vi "read_session.vi"(8 "error in (no error)":errorcluster caption="entrée d'erreur (pas d'erreur)", 11 "Python en entrée":refnum<class "Python.lvclass">) -> (0 "error out":errorcluster caption="sortie d'erreur", 2 "session":refnum<k35>, 3 "Python en sortie":refnum<class "Python.lvclass">)   [LabVIEW 2020, in "Python.lvclass"]
uses:
  Python.lvclass
  Python.lvclass/Python.ctl
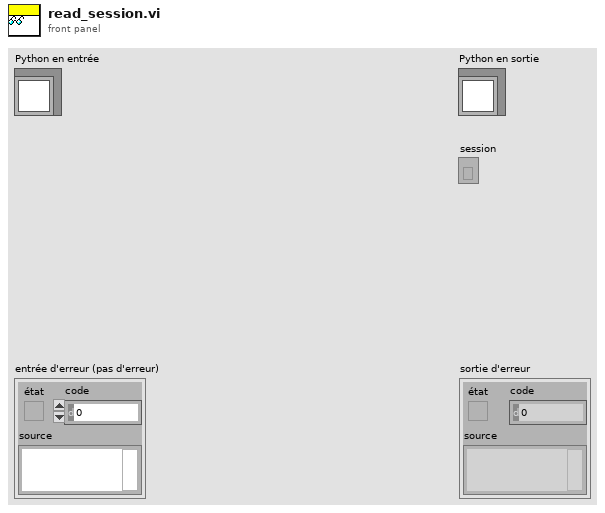
[diagram p1: front panel]
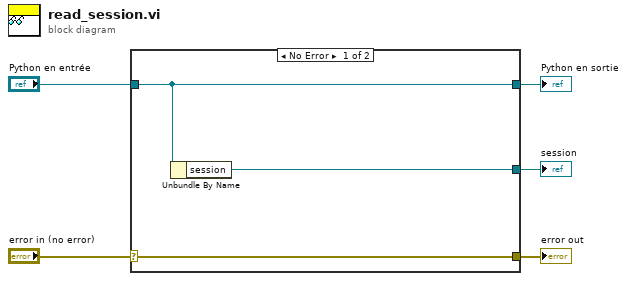
[diagram p0: block diagram]
diagram:
  n1 = case shown="No Error" "error in (no error)" {
    selector: "error in (no error)" -> [w8 w9]
    tunnel: [w8 w9] -> w4
    tunnel: [w7 w10] -> w2
    tunnel: "Python en entrée" -> [w7 w10]
    tunnel: [w6 _] -> w1
    frame No Error {
      n2 = Unbundle By Name(w7) -> ("session"=w6:refnum<k35>)
    }
    frame Error {
    }
  }
  "error out" <- w4
  "Python en sortie" <- w2
  "session" <- w1
